vi "Cache Transition Actions.vi"(0 "action queue in":refnum<queue>, 1 "TLB' Template in":refnum<class "TLB` - {TMPL}.lvclass">, 11 "error in (no error)":errorcluster) -> (3 "TLB' Template out":refnum<class "TLB` - {TMPL}.lvclass">, 15 "error out":errorcluster)   [LabVIEW 2016, in "TLB` Template.lvlib" / "TLB` - {TMPL}.lvclass"]
uses:
  TLB` - {TMPL}.lvclass
  TLB` - {TMPL}.lvclass/TLB` - {TMPL}.ctl
  Error Handler/TLB` Error Handler.lvclass/TLB` Error Handler.ctl
  Error Handler/accessors/Set Cache System Actions.vi
  Error Handler/accessors/Get Destination State.vi
  Actions/Actions.lvlib
  Error Handler/TLB` Error Handler.lvclass
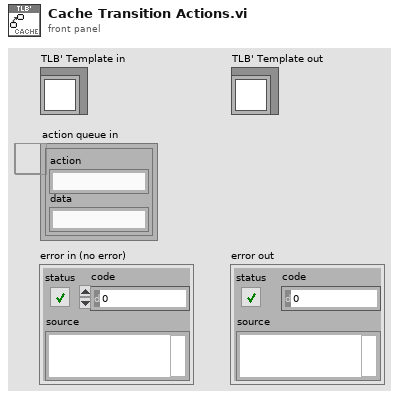
[diagram p1: front panel]
types:
  T1 = typedef "TLB` Template.lvlib/Actions.lvlib/System Action Element.ctl" = cluster{"action":string, "data":string}
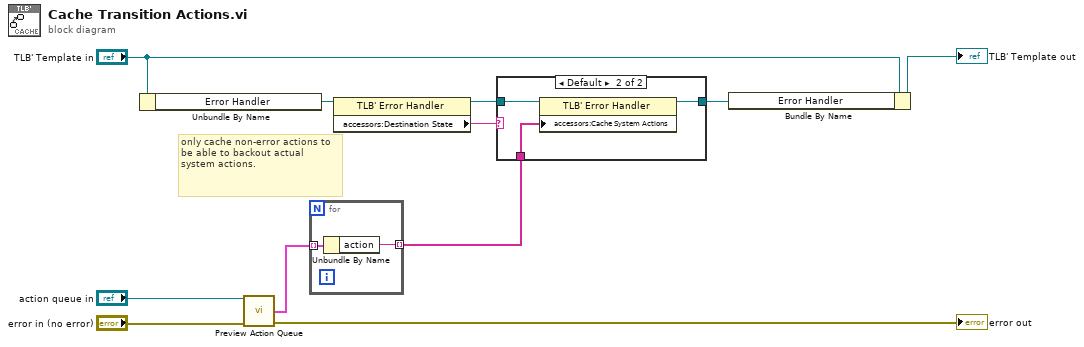
[diagram p0: block diagram]
diagram:
  # "only cache non-error actions to be able to backout actual system actions."
  n1 = Unbundle By Name("TLB' Template in") -> ("Error Handler"=w2:refnum<class "TLB` Error Handler.lvclass">)
  n2 = call "Preview Action Queue.vi"("action queue in"="action queue in", "error in"="error in (no error)") -> ("action elements"=w11:T1[], "error out"=→"error out":errorcluster)  [unwired: 11 in, 1 out]
  n3 = for {
    tunnel: w11 -> [w13] mode=indexing
    tunnel: [w12] -> w7 mode=indexing
    n4 = Unbundle By Name(w13) -> ("action"=w12:string)
  }
  n5 = property class="TLB' Error Handler"(reference=w2) -> (reference out=w9:refnum<class "TLB` Error Handler.lvclass">, "accessors:Destination State"=w8:string)  [unwired: 1 in, 1 out]
  n6 = case shown="Default" w8 {
    tunnel: w7 -> [_ w16]
    tunnel: w9 -> [w14 w17]
    tunnel: [w14 w15] -> w10
    frame "<Error>" {
    }
    frame Default {
      n7 = property class="TLB' Error Handler"(reference=w17, "accessors:Cache System Actions"=w16) -> (reference out=w15:refnum<class "TLB` Error Handler.lvclass">)  [unwired: 1 in, 1 out]
    }
  }
  n8 = Bundle By Name(cluster="TLB' Template in", "Error Handler"=w10) -> (→"TLB' Template out":refnum<class "TLB` - {TMPL}.lvclass">)
